vi "img_save.vi"() -> ()   [LabVIEW 2015]
uses:
  <vilib>/userdefined/High Color/IMAQdx.ctl
  <vilib>/vision/driver/NI_Vision_Acquisition_Software.lvlib
panel:
  in  "Path":path
  in  "Boolean":bool
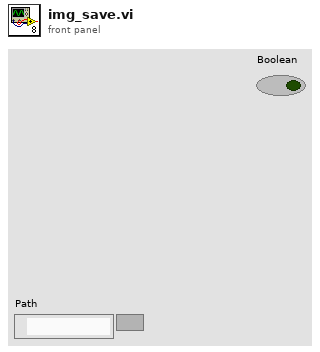
[diagram p1: front panel]
types:
  T1 = enum16{"open", "replace", "create", "open or create", "replace or create", "replace or create with confirmation"}
  T2 = typedef "Image Type" = u32
  T3 = typedef "IMAQdx.ctl" = refnum<k21>
  T4 = typedef "IMAQ Image.ctl" = refnum<image>
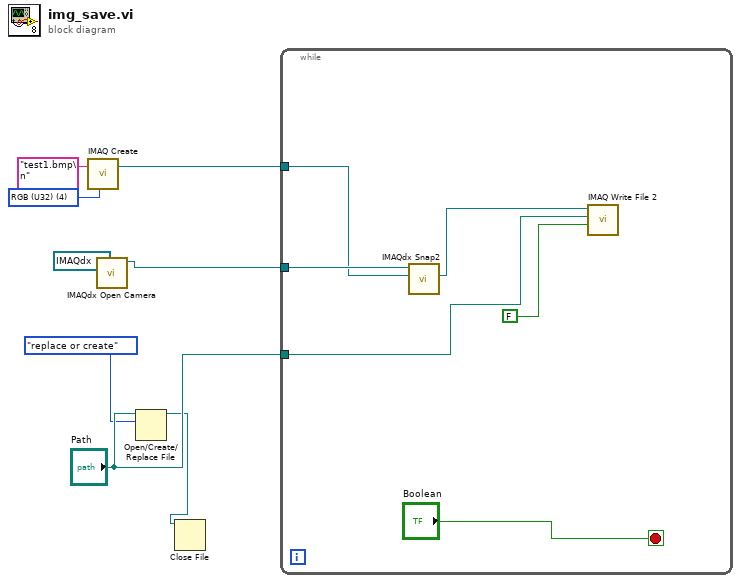
[diagram p0: block diagram]
diagram:
  w4 = T2 4 items=["Grayscale (U8)", "Grayscale (I16)", "Grayscale (SGL)", "Complex (CSG)", "RGB (U32)", "HSL (U32)", "RGB (U64)", "Grayscale (U16)"] ("Image Type")
  n1 = call "IMAQ Create"("Image Name"="test1.bmp\n", "Image Type"=w4) -> ("New Image"=w6:T4)  [unwired: 3 in, 1 out]
  n2 = call <vilib>:"IMAQdx Open Camera.vi"("Session In"=T3 "cam0") -> ("Session Out"=w7:T3)  [unwired: 9 in, 1 out]
  n3 = Open/Create/Replace File(file path (use dialog)="Path", operation (0:open)=T1."replace or create") -> (refnum out=w1:refnum<file>)  [unwired: 4 in, 2 out]
  n4 = Close File(refnum=w1) -> ()  [unwired: 1 in, 2 out]
  n5 = while {
    tunnel: w7 -> [w13]
    tunnel: w6 -> [w12]
    tunnel: "Path" -> [w9]
    stop <- "Boolean" stop-if-true
    n6 = call <vilib>:"IMAQdx Snap2.vi"("Image In"=w12, "Session In"=w13) -> ("Image Out"=w11:T4)  [unwired: 7 in, 2 out]
    n7 = call-poly "IMAQ Write File 2"("Compress? (N)"=FALSE, "File Path"=w9, "Image"=w11) -> ()  [unwired: 7 in, 2 out]
  }
